vi "DAQmx - Analyse(V)_SubVIs-某型振动实验台测试系统.vi"(8 "Error In":errorcluster, 11 "Vibration Waveform":waveform(dbl)[](array[waveform])) -> (0 "Error Out":errorcluster, 3 "Display Info":T1)   [LabVIEW 2011]
uses:
  <vilib>/Analysis/5stat.llb/RMS (DBL).vi
  <vilib>/Analysis/NI_AALPro.lvlib
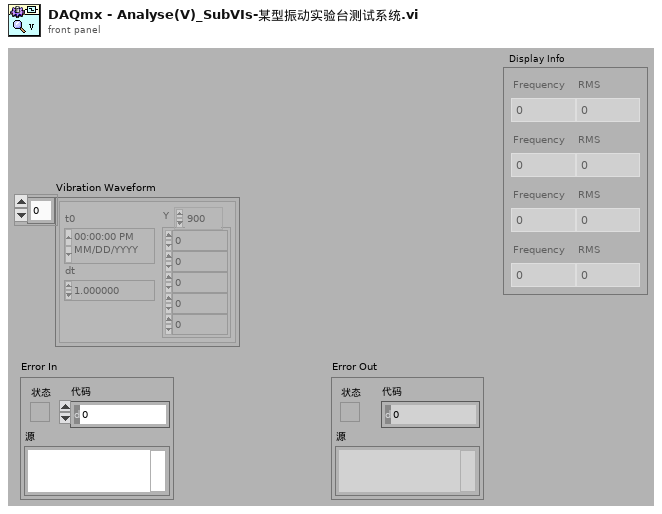
[diagram p1: front panel]
types:
  T1 = typedef "Display Information_Ctrls-某型振动实验台测试系统.ctl" = cluster{"Frequency":dbl, "RMS":dbl}[]
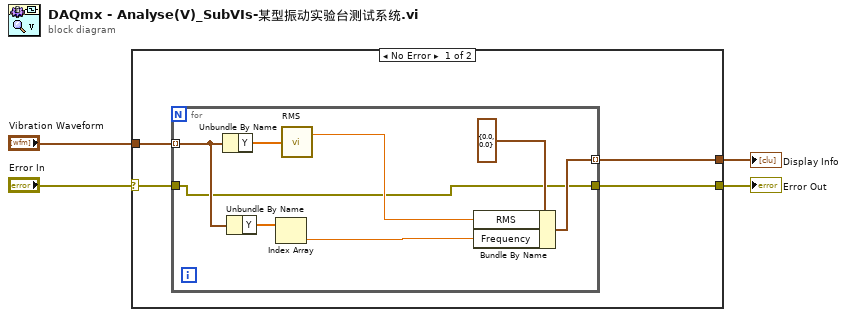
[diagram p0: block diagram]
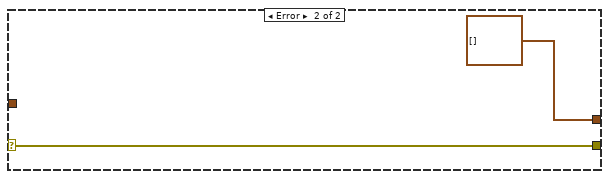
[diagram p2: hidden frame]
diagram:
  n1 = case shown="No Error" "Error In" {
    selector: "Error In" -> [w7 w18]
    tunnel: [w6 w18] -> w3
    tunnel: "Vibration Waveform" -> [w8 _]
    tunnel: [w5 cluster{"Frequency":dbl, "RMS":dbl}[] []] -> w1
    frame No Error {
      n2 = for {
        tunnel: [w16] -> w5 mode=indexing
        tunnel: w8 -> [w12] mode=indexing
        tunnel: w7 -> [w9]
        tunnel: [w9] -> w6
        n3 = Unbundle By Name(w12) -> ("Y"=w14:dbl[])
        n4 = Unbundle By Name(w12) -> ("Y"=w11:dbl[])
        n5 = Index Array(array=w11) -> (element=w10:dbl)  [unwired: 1 in]
        n6 = call-poly <vilib>:"RMS.vi"("X"=w14) -> ("rms value"=w15:dbl)  [unwired: 1 out]
        n7 = Bundle By Name(cluster=cluster{"Frequency":dbl, "RMS":dbl} {"Frequency"=0.0, "RMS"=0.0} ("元素"), "RMS"=w15, "Frequency"=w10) -> (w16:cluster{"Frequency":dbl, "RMS":dbl})
      }
    }
    frame Error {
    }
  }
  "Error Out" <- w3
  "Display Info" <- w1
